vi "STD Next Check.vi"(8 "에러 입력":errorcluster caption="에러 입력(에러 없음)", 10 "Data in":string[][](array[string]), 11 "기준기리스트 참조 입력":refnum<vi>) -> (0 "에러 출력":errorcluster, 2 "Data out":string[][](array[string]), 3 "기준기리스트 참조 출력":refnum<vi>)   [LabVIEW 2020]
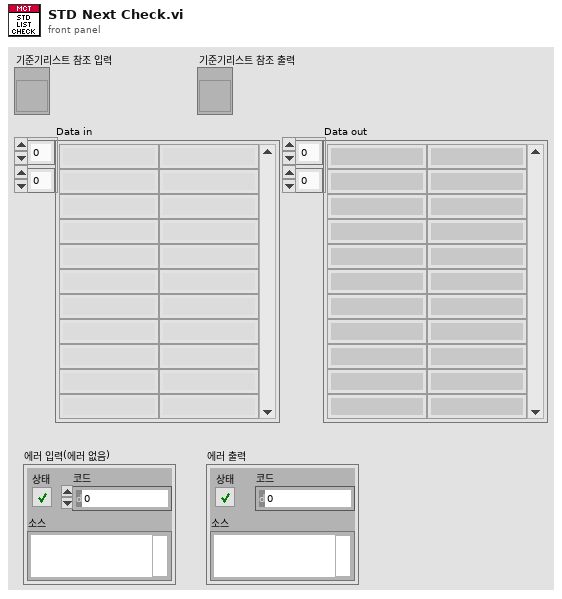
[diagram p1: front panel]
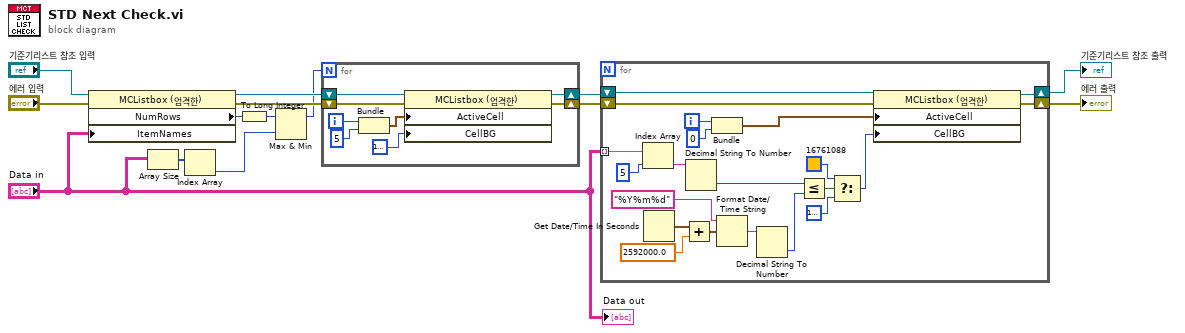
[diagram p0: block diagram]
diagram:
  n1 = property on="프로퍼티 노드" class="MCListbox (엄격한)"(reference="기준기리스트 참조 입력", error in="에러 입력", "ItemNames"="Data in") -> (reference out=w7:refnum<vi>, error out=w9:errorcluster, "NumRows"=w5:u32)
  n2 = Array Size(array="Data in") -> (size(s)=w6:i32[])
  n3 = Index Array(array=w6) -> (element=w3:i32)  [unwired: 1 in]
  n4 = To Long Integer(number=w5) -> (32bit integer=w2:i32)
  n5 = Max & Min(x=w2, y=w3) -> (max(x,y)=w4:i32)  [unwired: 1 out]
  n6 = for {
    N: w4 -> [_]
    shift-right: [w22] -> w12
    shift-left: w9 -> [w20]
    shift-right: [w21] -> w11
    shift-left: w7 -> [w19]
    i -> [w16]
    n7 = Bundle(w16, 5) -> (w17:cluster{i32, i32})  [unwired: 1 in]
    n8 = property on="프로퍼티 노드" class="MCListbox (엄격한)"(reference=w19, error in=w20, "ActiveCell"=w17, "CellBG"=u32 16777225) -> (reference out=w21:refnum<vi>, error out=w22:errorcluster)
  }
  n9 = for {
    tunnel: "Data in" -> [w43] mode=indexing
    shift-right: [w32] -> w13
    shift-left: w11 -> [w33]
    shift-right: [w30] -> w14
    shift-left: w12 -> [w31]
    i -> [w28]
    n10 = Index Array(array=w43, index=5 ("인덱스")) -> (element=w41:string)
    n11 = Get Date/Time In Seconds() -> (seconds since 1Jan1904=w40:timestamp)
    n12 = Add(x=w40, y=2592000.0) -> (x+y=w38:timestamp)
    n13 = Decimal String To Number(string=w41) -> (number=w35:i32)  [unwired: 2 in, 1 out]
    n14 = Bundle(w28, 0) -> (w29:cluster{i32, i32})  [unwired: 1 in]
    n15 = Format Date/Time String(time format string (%c)="%Y%m%d" ("시간 포맷 문자열 (%c)"), seconds (now)=w38) -> (date/time string=w37:string)  [unwired: 1 in]
    n16 = Decimal String To Number(string=w37) -> (number=w34:i32)  [unwired: 2 in, 1 out]
    n17 = Less Or Equal?(x=w35, y=w34) -> (x <= y?=w26:bool)
    n18 = Select(t=u32 16761088, s=w26, f=u32 16777225) -> (s? t:f=w23:u32)
    n19 = property on="프로퍼티 노드" class="MCListbox (엄격한)"(reference=w33, error in=w31, "ActiveCell"=w29, "CellBG"=w23) -> (reference out=w32:refnum<vi>, error out=w30:errorcluster)
  }
  "에러 출력" <- w14
  "기준기리스트 참조 출력" <- w13
  "Data out" <- "Data in"
